vi "junk01.vi"() -> ()   [LabVIEW 2013]
uses:
  C:/Program Files (x86)/National Instruments/LabVIEW 2013/vi.lib/ULx/ULx_LV.dll
  <vilib>/DAQmx/create/channels.llb/DAQmx Create Channel (AI-Voltage-Basic).vi
panel:
  in  "i/o task in":refnum<k24>
  in  "error in (no error)":errorcluster
  in  "taskType":i32(ring) items=["AnalogInput", "AnalogOutput", "CompoundInput", "CompoundOutput", "CounterInput", "CounterOutput", "DigitalInput", "DigitalOutput", "TemperatureInput"]
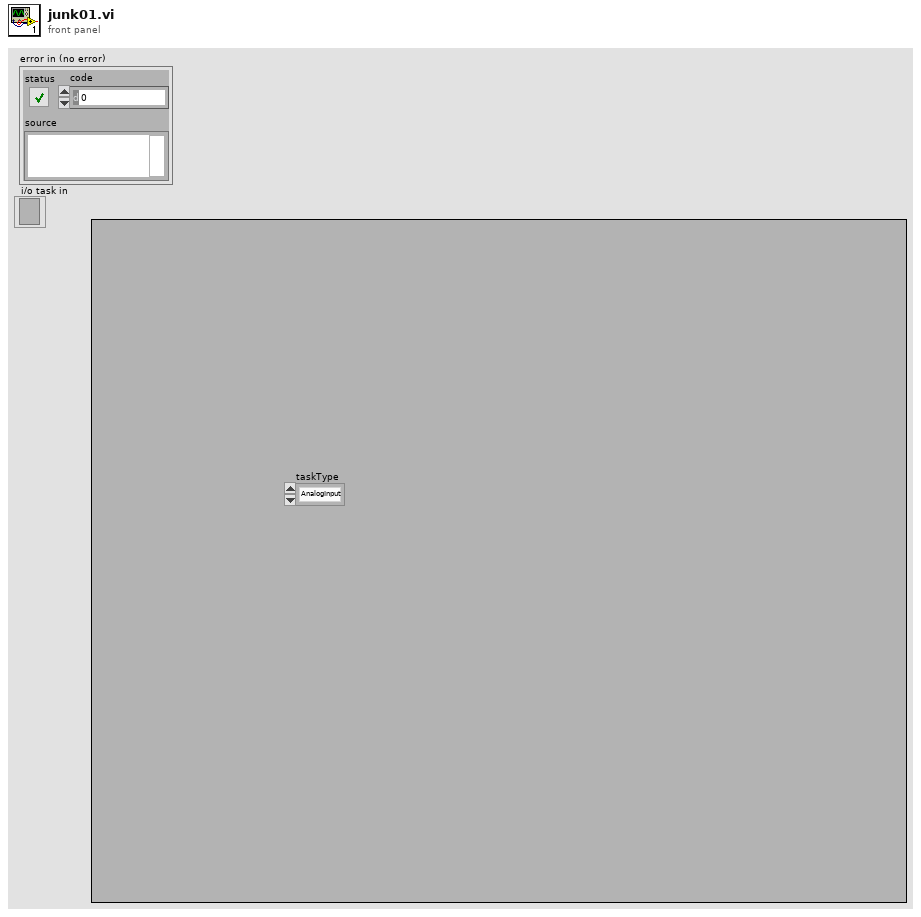
[diagram p1: front panel]
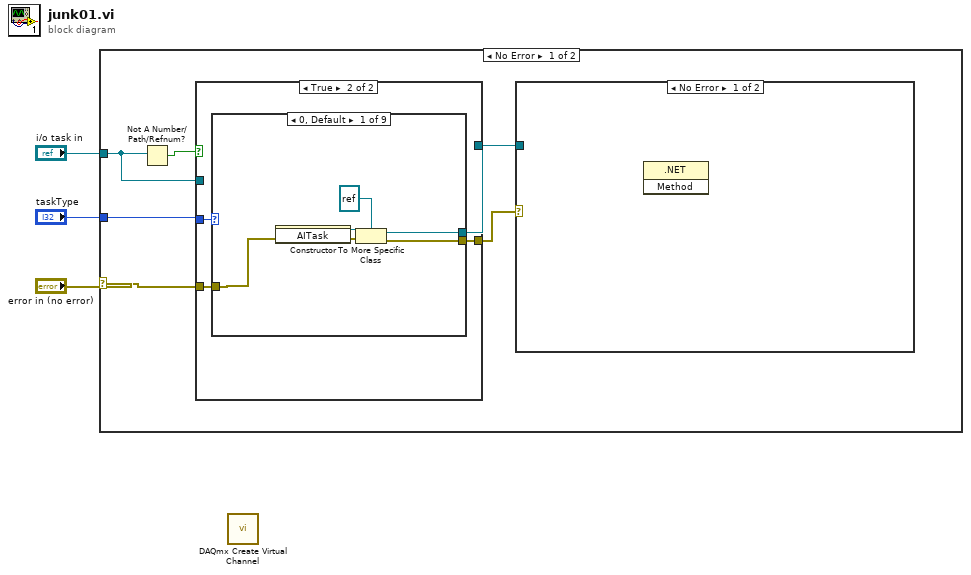
[diagram p0: block diagram]
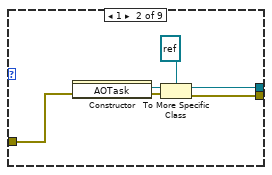
[diagram p3: hidden frame]
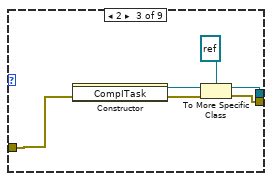
[diagram p4: hidden frame]
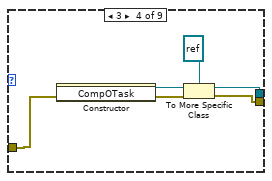
[diagram p5: hidden frame]
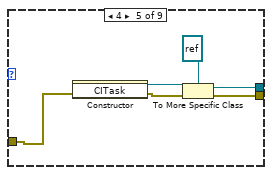
[diagram p6: hidden frame]
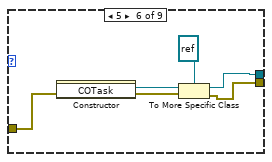
[diagram p7: hidden frame]
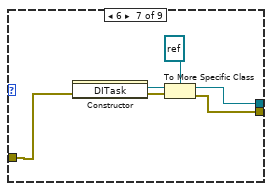
[diagram p8: hidden frame]
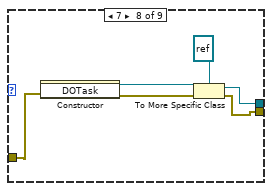
[diagram p9: hidden frame]
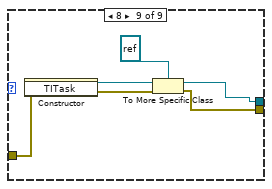
[diagram p10: hidden frame]
diagram:
  n1 = case shown="No Error" "error in (no error)" {
    selector: "error in (no error)" -> [w7 _]
    tunnel: "i/o task in" -> [w5 _]
    tunnel: "taskType" -> [w4 _]
    frame No Error {
      n2 = Not A Number/Path/Refnum?(number/path/refnum=w5) -> (NaN/Path/Refnum?=w6:bool)
      n3 = case shown="True" w6 {
        tunnel: w4 -> [_ w13]
        tunnel: [_ w12] -> w9
        tunnel: [_ w11] -> w8
        tunnel: w7 -> [_ w10]
        tunnel: w5 -> [_ _]
        frame False {
        }
        frame True {
          n4 = case shown="0, Default" w13 {
            tunnel: w10 -> [w16 w22 w28 w34 w41 w46 w52 w58 w64]
            tunnel: [w15 w21 w27 w33 w40 w45 w51 w56 w63] -> w12
            tunnel: [w14 w20 w26 w32 w38 w44 w50 w57 w62] -> w11
            frame 0, Default {
              n5 = constructor class="AITask"(error in=w16) -> (reference out=w18:refnum<k24>, error out=w17:errorcluster)  [unwired: 2 in, 1 out]
              n6 = To More Specific Class(target class=refnum<k24> refnum (".NET Refnum"), reference=w18, error in=w17) -> (specific class reference=w15:refnum<k24>, error out=w14:errorcluster)
            }
            frame 1 {
              n7 = constructor class="AOTask"(error in=w22) -> (reference out=w24:refnum<k24>, error out=w23:errorcluster)  [unwired: 2 in, 1 out]
              n8 = To More Specific Class(target class=refnum<k24> refnum (".NET Refnum"), reference=w24, error in=w23) -> (specific class reference=w21:refnum<k24>, error out=w20:errorcluster)
            }
            frame 2 {
              n9 = constructor class="CompITask"(error in=w28) -> (reference out=w30:refnum<k24>, error out=w31:errorcluster)  [unwired: 2 in, 1 out]
              n10 = To More Specific Class(target class=refnum<k24> refnum (".NET Refnum"), reference=w30, error in=w31) -> (specific class reference=w27:refnum<k24>, error out=w26:errorcluster)
            }
            frame 3 {
              n11 = constructor class="CompOTask"(error in=w34) -> (reference out=w36:refnum<k24>, error out=w37:errorcluster)  [unwired: 2 in, 1 out]
              n12 = To More Specific Class(target class=refnum<k24> refnum (".NET Refnum"), reference=w36, error in=w37) -> (specific class reference=w33:refnum<k24>, error out=w32:errorcluster)
            }
            frame 4 {
              n13 = constructor class="CITask"(error in=w41) -> (reference out=w42:refnum<k24>, error out=w39:errorcluster)  [unwired: 2 in, 1 out]
              n14 = To More Specific Class(target class=refnum<k24> refnum (".NET Refnum"), reference=w42, error in=w39) -> (specific class reference=w40:refnum<k24>, error out=w38:errorcluster)
            }
            frame 5 {
              n15 = constructor class="COTask"(error in=w46) -> (reference out=w48:refnum<k24>, error out=w49:errorcluster)  [unwired: 2 in, 1 out]
              n16 = To More Specific Class(target class=refnum<k24> refnum (".NET Refnum"), reference=w48, error in=w49) -> (specific class reference=w45:refnum<k24>, error out=w44:errorcluster)
            }
            frame 6 {
              n17 = constructor class="DITask"(error in=w52) -> (reference out=w54:refnum<k24>, error out=w55:errorcluster)  [unwired: 2 in, 1 out]
              n18 = To More Specific Class(target class=refnum<k24> refnum (".NET Refnum"), reference=w54, error in=w55) -> (specific class reference=w51:refnum<k24>, error out=w50:errorcluster)
            }
            frame 7 {
              n19 = constructor class="DOTask"(error in=w58) -> (reference out=w60:refnum<k24>, error out=w61:errorcluster)  [unwired: 2 in, 1 out]
              n20 = To More Specific Class(target class=refnum<k24> refnum (".NET Refnum"), reference=w60, error in=w61) -> (specific class reference=w56:refnum<k24>, error out=w57:errorcluster)
            }
            frame 8 {
              n21 = constructor class="TITask"(error in=w64) -> (reference out=w67:refnum<k24>, error out=w66:errorcluster)  [unwired: 2 in, 1 out]
              n22 = To More Specific Class(target class=refnum<k24> refnum (".NET Refnum"), reference=w67, error in=w66) -> (specific class reference=w63:refnum<k24>, error out=w62:errorcluster)
            }
          }
        }
      }
      n23 = case shown="No Error" w8 {
        tunnel: w9 -> [_ _]
        frame No Error {
          n24 = invoke class=".NET" method=#-1() -> ()  [unwired: 3 in, 3 out]
        }
        frame Error {
        }
      }
    }
    frame Error {
    }
  }
  n25 = call-poly <vilib>:"DAQmx Create Virtual Channel.vi"() -> ()  [unwired: 14 in, 2 out]
